vi "Hang Immediate.vi"(9 "Ratchet":T1, 10 "Angle":T1, 11 "Setpoint":dbl) -> ()   [LabVIEW 2019]
uses:
  <vilib>/Rock Robotics/WPI/Solenoid/WPI_SolenoidValue.ctl
  Implementation/Hang Operations.ctl
  Implementation/Hang Setpoints.ctl
  <vilib>/Rock Robotics/WPI/Framework/Completion Status.ctl
  <vilib>/Rock Robotics/WPI/Framework/Completion Notifier.ctl
  <vilib>/Rock Robotics/WPI/Framework/Command Status Info.ctl
panel:
  in  "Description":string
  out "Command Info Out":T2
  in  "Command Info In":T2
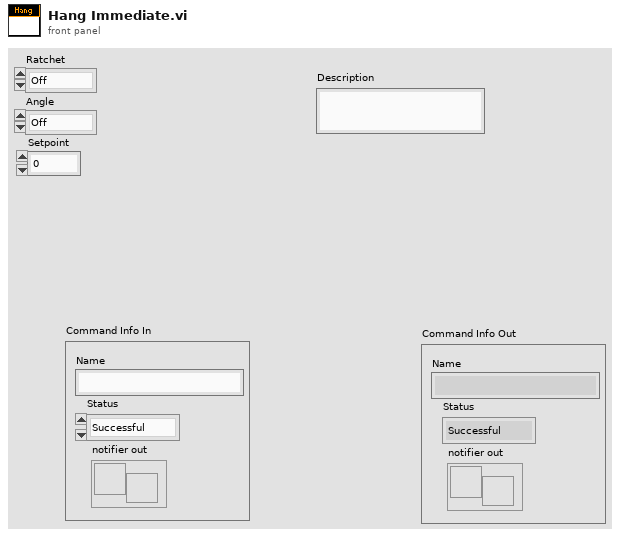
[diagram p1: front panel]
types:
  T1 = typedef "WPI_SolenoidValue.ctl" = enum16{"Off", "On", "Forward", "Reverse"}
  T2 = typedef "Command Status Info.ctl" = cluster{"Name":string, "Status":T3, "notifier out":T4}
  T3 = typedef "Completion Status.ctl" = enum16{"Successful", "Aborted", "Incomplete"}
  T4 = typedef "Completion Notifier.ctl" = refnum<notifier>
  T5 = typedef "Hang Setpoints.ctl" = cluster{"Operation":T6, "Ratchet":T1, "Angle":T1, "Setpoint":dbl}
  T6 = typedef "Hang Operations.ctl" = enum16{"Reserve", "Read Current", "Immediate"}
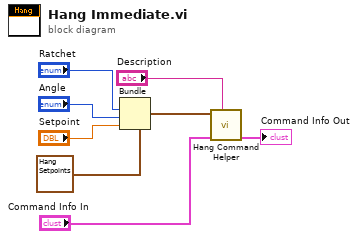
[diagram p0: block diagram]
diagram:
  n1 = Bundle(cluster=T5 {"Operation"=enum."Immediate", "Ratchet"=enum."Off", "Angle"=enum."Off", "Setpoint"=0.0} ("SubSystem Data"), "Ratchet"="Ratchet", "Angle"="Angle", "Setpoint"="Setpoint") -> (w4:T5)  [unwired: 1 in]
  n2 = call "Hang Command Helper.vi"("Description"="Description", "Command Info In"="Command Info In", "SubSystem Data"=w4) -> ("Command Info Out"=→"Command Info Out":T2)  [unwired: 6 in, 2 out]
